vi "Lab1_4.vi"() -> ()   [LabVIEW 2021]
panel:
  out "Array":dbl[][](array[numeric])
  out "Third Row Fifth Column":dbl
  out "Third Row":dbl[](array[numeric])
  out "Second Column":dbl[](array[numeric])
  in  "Columns":i32=80
  in  "Rows":i32=80
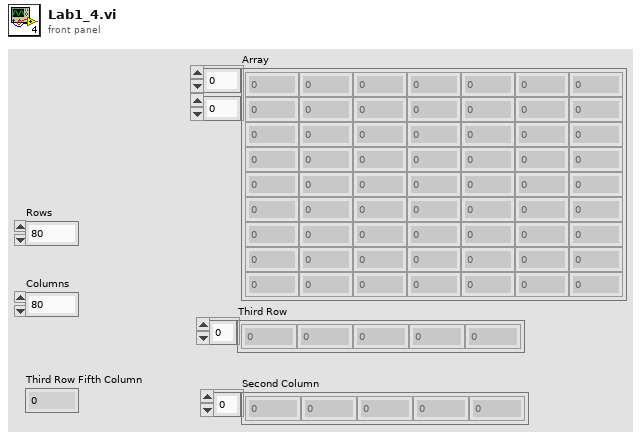
[diagram p1: front panel]
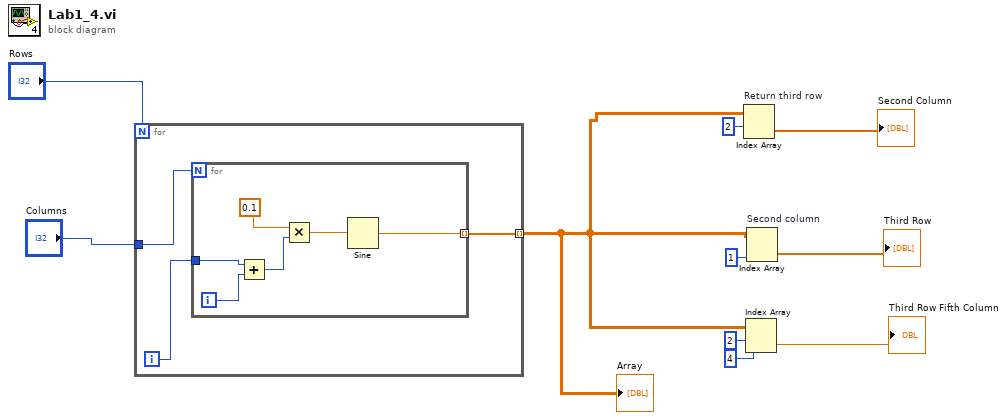
[diagram p0: block diagram]
diagram:
  n1 = for {
    N: "Rows" -> [_]
    tunnel: "Columns" -> [w13]
    tunnel: [w11] -> w1 mode=indexing
    i -> [w12]
    n2 = for {
      N: w13 -> [_]
      tunnel: w12 -> [w19]
      tunnel: [w14] -> w11 mode=indexing
      i -> [w18]
      n3 = Add(x=w19, y=w18) -> (x+y=w17:i32)
      n4 = Multiply(x=0.1, y=w17) -> (x*y=w16:dbl)
      n5 = Sine(x=w16) -> (sin(x)=w14:dbl)
    }
  }
  "Array" <- w1
  n6 = Index Array "Return third row"(array=w1, index (row)=2) -> (element=→"Second Column":dbl[])  [unwired: 1 in]
  n7 = Index Array(array=w1, index (row)=2, index (col)=4 ("disabled index (col)")) -> (element=→"Third Row Fifth Column":dbl)
  n8 = Index Array "Second column"(array=w1, index (col)=1 ("disabled index (col)")) -> (element=→"Third Row":dbl[])  [unwired: 1 in]
